vi "649FinalN.vi"() -> ()   [LabVIEW 2023]
uses:
  <vilib>/Utility/file.llb/Write Delimited Spreadsheet (string).vi
panel:
  in  "Button 2":bool
  in  "Button 1":bool
  out "?":string[](array[string])
  in  "?":bool
  out "?":i32[][](array[numeric])
  # "6@49"
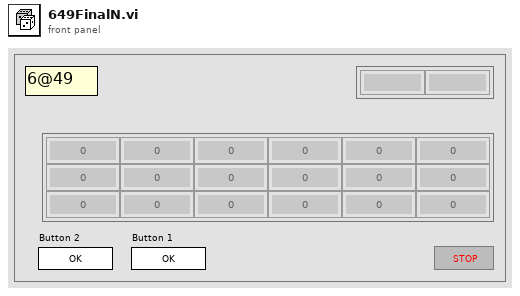
[diagram p1: front panel]
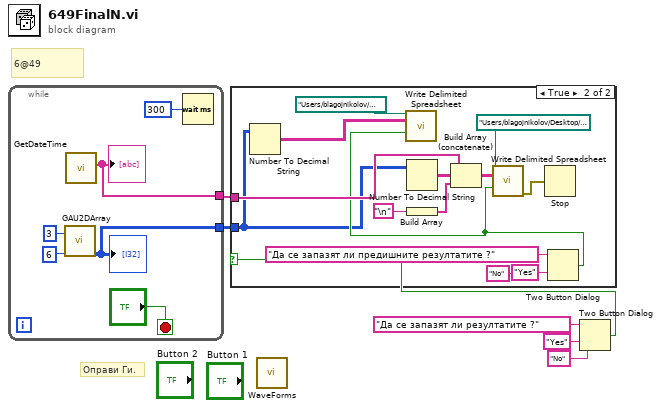
[diagram p0: block diagram]
diagram:
  # "Оправи Ги."
  # "6@49"
  n1 = while {
    tunnel: [w9] -> w5
    tunnel: [w10] -> w6
    stop <- "?" stop-if-true
    n2 = call "GAU2DArray.vi"("Colums"=6, "Rows"=3) -> ("2D Double Array"=w9:i32[][])  [unwired: 8 in, 1 out]
    "?" <- w9
    n3 = call "GetDateTime.vi"() -> (2:w10:string[])  [unwired: 11 in]
    "?" <- w10
    n4 = Wait (ms)(milliseconds to wait=u32 300) -> ()  [unwired: 1 out]
  }
  n5 = call "WaveForms.vi"() -> ()  [unwired: 8 in, 3 out]
  n6 = Two Button Dialog(message="Да се запазят ли резултатите ?", 1:"No" ("F button name (\"Cancel\")"), 2:"Yes" ("T button name (\"OK\")")) -> (T button?=w3:bool)
  n7 = case shown="True" w3 {
    tunnel: w6 -> [_ w25]
    tunnel: w5 -> [_ w14]
    frame False {
    }
    frame True {
      n8 = Number To Decimal String(number=w14) -> (decimal integer string=w13:string[][])  [unwired: 1 in]
      n9 = Number To Decimal String(number=w14) -> (decimal integer string=w24:string[][])  [unwired: 1 in]
      n10 = Build Array "Build Array"("\n") -> (w22:string[])
      n11 = Build Array (concatenate)(w25, w24, w22) -> (w26:string[][])
      n12 = Two Button Dialog(message="Да се запазят ли предишните резултатите ?", 1:"No" ("F button name (\"Cancel\")"), 2:"Yes" ("T button name (\"OK\")")) -> (T button?=w15:bool)
      n13 = call-poly <vilib>:"Write Delimited Spreadsheet.vi"("file path (dialog if empty)"=path "/Users/blagojnikolov/Desktop/@tmp/archive.txt", "2D data"=w13, "append to file? (new file:F)"=w15) -> ()  [unwired: 11 in, 2 out]
      n14 = call-poly <vilib>:"Write Delimited Spreadsheet.vi"("file path (dialog if empty)"=path "/Users/blagojnikolov/Desktop/@tmp/toto.txt" ("file path"), "2D data"=w26, "append to file? (new file:F)"=w15) -> ("error out"=w20:errorcluster)  [unwired: 11 in, 1 out]
      n15 = Stop(stop? (T)=w20) -> ()
    }
  }
